vi "Przelicz ROS-a.vi"(11 "value 2":T1) -> (3 "output cluster":cluster{dbl, dbl})   [LabVIEW 2015]
panel:
  out "axes":sgl[](array[numeric])
  out "buttons":i32[](array[numeric])
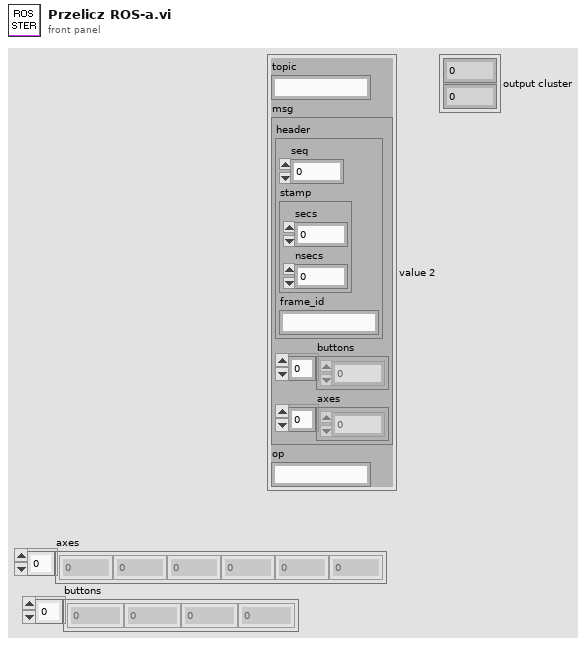
[diagram p1: front panel]
types:
  T1 = cluster{"topic":string, "msg":cluster{"header":cluster{"seq":u32, "stamp":cluster{"secs":u32, "nsecs":i32}, "frame_id":string}, "buttons":i32[], "axes":sgl[]}, "op":string}
  T2 = cluster{"header":cluster{"seq":u32, "stamp":cluster{"secs":u32, "nsecs":i32}, "frame_id":string}, "buttons":i32[], "axes":sgl[]}
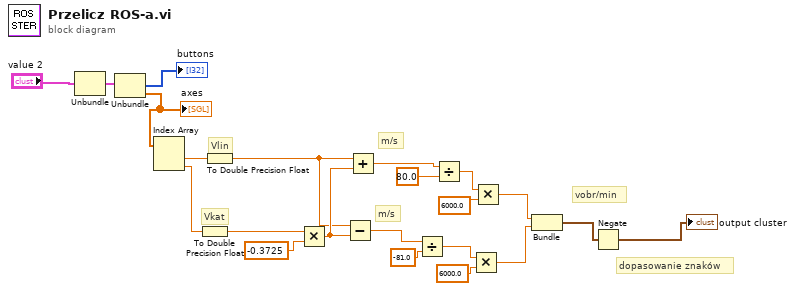
[diagram p0: block diagram]
diagram:
  # "dopasowanie znaków"
  # "vobr/min"
  # "m/s"
  # "m/s"
  # "Vkat"
  # "Vlin"
  n1 = Unbundle("value 2") -> ("msg"=w20:T2)  [unwired: 2 out]
  n2 = Unbundle(w20) -> ("buttons"=→"buttons":i32[], "axes"=w17:sgl[])  [unwired: 1 out]
  "axes" <- w17
  n3 = Index Array(array=w17) -> (element #1=w15:sgl, element #2=w16:sgl)  [unwired: 2 in]
  n4 = To Double Precision Float(number=w16) -> (double precision float=w5:dbl)
  n5 = To Double Precision Float(number=w15) -> (double precision float=w11:dbl)
  n6 = Multiply(x=w5, y=-0.3725) -> (x*y=w21:dbl)
  n7 = Subtract(x=w11, y=w21) -> (x-y=w9:dbl)
  n8 = Add(x=w11, y=w21) -> (x+y=w10:dbl)
  n9 = Divide(x=w9, y=-81.0) -> (x/y=w7:dbl)
  n10 = Divide(x=w10, y=80.0) -> (x/y=w8:dbl)
  n11 = Multiply(x=w7, y=6000.0) -> (x*y=w3:dbl)
  n12 = Multiply(x=w8, y=6000.0) -> (x*y=w4:dbl)
  n13 = Bundle(w4, w3) -> (w1:cluster{dbl, dbl})  [unwired: 1 in]
  n14 = Negate(x=w1) -> (-x=→"output cluster":cluster{dbl, dbl})
